vi "Determine Condition.vi"(8 "error in (no error)":errorcluster, 11 "RMS":dbl) -> (0 "error out":errorcluster, 3 "Condition":i32)   [LabVIEW 2026, in "Acquisition.lvlib"]
uses:
  Acquisition.lvlib
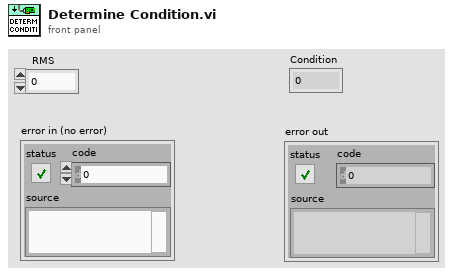
[diagram p1: front panel]
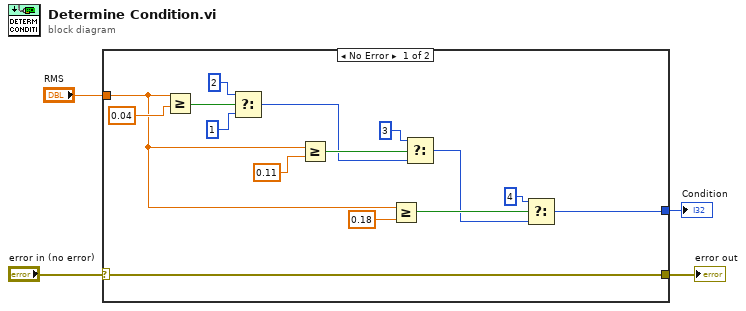
[diagram p0: block diagram]
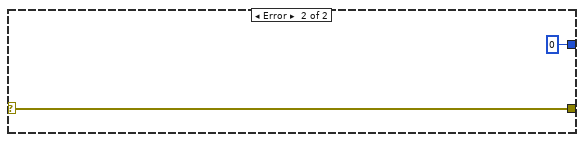
[diagram p2: hidden frame]
diagram:
  n1 = case shown="No Error" "error in (no error)" {
    selector: "error in (no error)" -> [w9 w21]
    tunnel: "RMS" -> [w14 _]
    tunnel: [w10 0] -> w1
    tunnel: [w9 w21] -> w2
    frame No Error {
      n2 = Greater Or Equal?(x=w14, y=0.04 ("x")) -> (x >= y?=w19:bool)
      n3 = Select(t=2, s=w19, f=1) -> (s? t:f=w16:i32)
      n4 = Greater Or Equal?(x=w14, y=0.11 ("x")) -> (x >= y?=w18:bool)
      n5 = Greater Or Equal?(x=w14, y=0.18 ("x")) -> (x >= y?=w12:bool)
      n6 = Select(t=3, s=w18, f=w16) -> (s? t:f=w11:i32)
      n7 = Select(t=4, s=w12, f=w11) -> (s? t:f=w10:i32)
    }
    frame Error {
    }
  }
  "error out" <- w2
  "Condition" <- w1
